vi "告警接口-告警存储-交互.vi"(11 "map in":T1) -> (3 "data":T2)   [LabVIEW 2016, in "Alarm interface.lvlib"]
uses:
  Alarm interface.lvlib
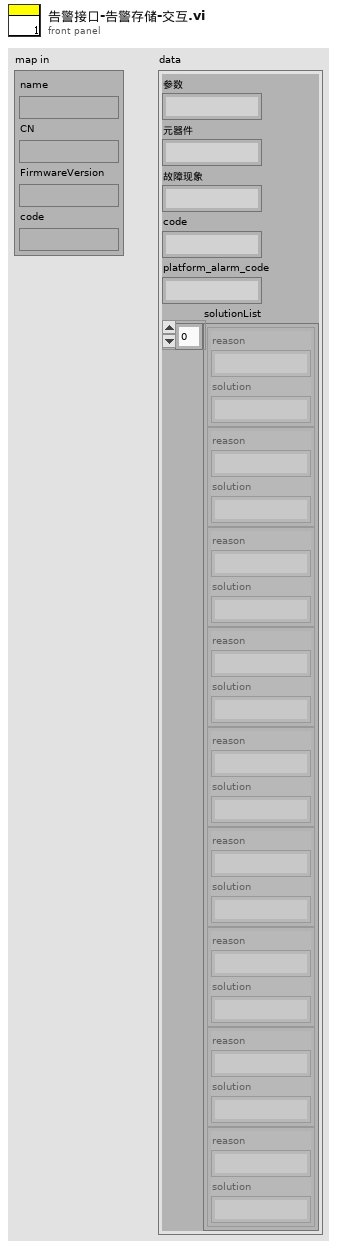
[diagram p1: front panel]
types:
  T1 = typedef "Alarm interface.lvlib/map in.ctl" = cluster{"name":string, "CN":string, "FirmwareVersion":string, "code":string}
  T2 = typedef "Alarm interface.lvlib/报警短信语音交互.ctl" = cluster{"参数":string, "元器件":string, "故障现象":string, "code":string, "platform_alarm_code":string, "solutionList":cluster{"reason":string, "solution":string}[]}
  T3 = typedef "Alarm interface.lvlib/map out.ctl" = cluster{"componentParent":string, "componentName":string, "equipVersion":string, "ipcAlarmCode":string, "faultPhenomenon":string}
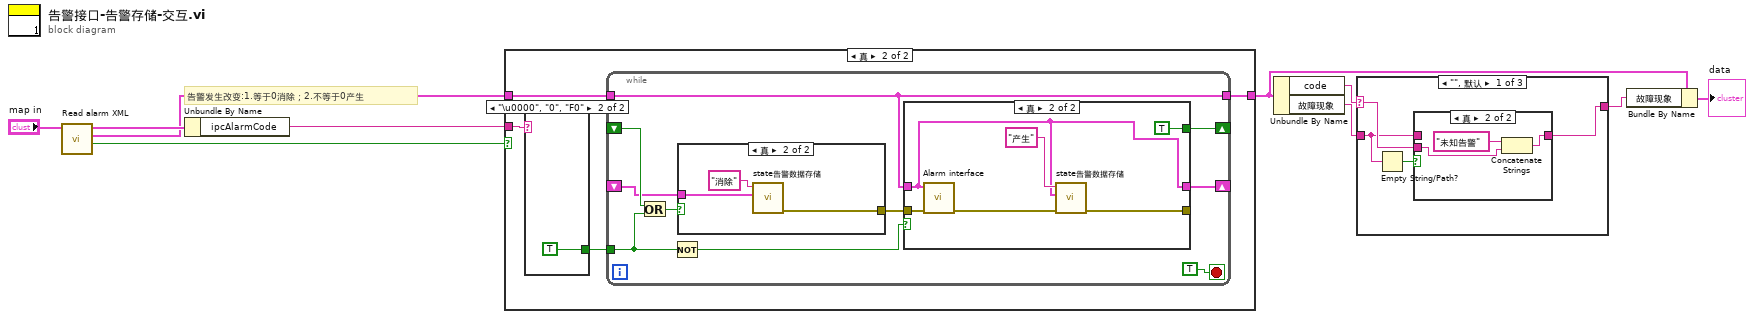
[diagram p0: block diagram]
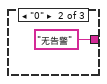
[diagram p7: hidden frame]
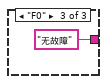
[diagram p8: hidden frame]
diagram:
  # "告警发生改变:1.等于0消除；2.不等于0产生"
  n1 = call "Read alarm XML.vi"("map in"="map in") -> ("map out"=w10:T3, "data"=w2:T2, "change?"=w4:bool)  [unwired: 7 in]
  n2 = Unbundle By Name(w10) -> ("ipcAlarmCode"=w3:string)
  n3 = case shown="真" w4 {
    tunnel: w3 -> [_ w15]
    tunnel: w2 -> [w11 w13]
    tunnel: [w11 w12] -> w1
    frame False {
    }
    frame True {
      n4 = case shown="\"\", \"0\", \"F0\"" w15 {
        tunnel: [_ TRUE] -> w14
        frame "假", Default {
        }
        frame "\u0000", "0", "F0" {
        }
      }
      n5 = while {
        shift-right: [w20] -> _
        shift-left: _ -> [w25]
        tunnel: w14 -> [w23]
        tunnel: w13 -> [w17]
        shift-right: [w18] -> _
        shift-left: _ -> [w19]
        tunnel: [w17] -> w12
        stop <- TRUE stop-if-true
        n6 = Or(x=w25, y=w23) -> (x .or. y?=w24:bool)
        n7 = Not(x=w23) -> (.not. x?=w22:bool)
        n8 = case shown="真" w24 {
          tunnel: [_ w35] -> w21
          tunnel: w19 -> [_ w34]
          frame False {
          }
          frame True {
            n9 = call "state告警数据存储.vi"("data"=w34, "state"="消除") -> ("错误输出"=w35:errorcluster)  [unwired: 9 in]
          }
        }
        n10 = case shown="真" w22 {
          tunnel: w21 -> [_ w33]
          tunnel: w17 -> [w27 w28]
          tunnel: [_ w30] -> _
          tunnel: [_ TRUE] -> w20
          tunnel: [w27 w28] -> w18
          frame False {
          }
          frame True {
            n11 = call "Alarm interface.vi"("错误输入（无错误）"=w33, "簇"=w28) -> ("错误输出"=w31:errorcluster)  [unwired: 9 in]
            n12 = call "state告警数据存储.vi"("错误输入（无错误）"=w31, "data"=w28, "state"="产生") -> ("错误输出"=w30:errorcluster)  [unwired: 8 in]
          }
        }
      }
    }
  }
  n13 = Unbundle By Name(w1) -> ("code"=w9:string, "故障现象"=w8:string)
  n14 = case shown="\"\", 默认" w9 {
    selector: w9 -> [w39 _ _]
    tunnel: w8 -> [w37 _ _]
    tunnel: [w38 "无告警" "无故障"] -> w7
    frame "", Default {
      n15 = Empty String/Path?(string/path=w37) -> (empty?=w40:bool)
      n16 = case shown="真" w40 {
        tunnel: w39 -> [_ w43]
        tunnel: [w41 w42] -> w38
        tunnel: w37 -> [w41 _]
        frame False {
        }
        frame True {
          n17 = Concatenate Strings("未知告警", w43) -> (w42:string)
        }
      }
    }
    frame "0" {
    }
    frame "F0" {
    }
  }
  n18 = Bundle By Name(cluster=w1, "故障现象"=w7) -> (→"data":T2)
